vi "4 Axis - Wait for Arrival.vi"(4 "error in (no error)":errorcluster, 7 "Controller Reference In":refnum<k7>) -> (0 "error out":errorcluster, 3 "Controller Reference out":refnum<k7>)   [LabVIEW 2015]
doc: "Waits for all 4 Axis to arrive at their set Target Positions."
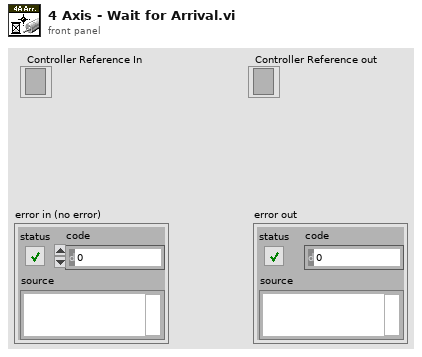
[diagram p1: front panel]
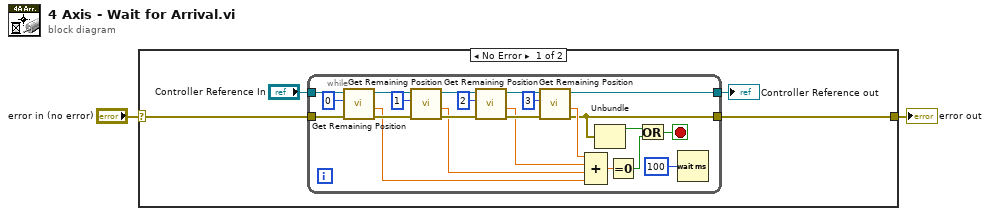
[diagram p0: block diagram]
diagram:
  n1 = case shown="No Error" "error in (no error)" {
    selector: "error in (no error)" -> [w3 w30]
    tunnel: [w4 w30] -> w2
    frame No Error {
      n2 = while {
        tunnel: "Controller Reference In" -> [w29]
        tunnel: [w17] -> w5
        tunnel: w3 -> [w28]
        tunnel: [w11] -> w4
        stop <- w8 stop-if-true
        n3 = call "Get Remaining Position.vi"("error in (no error)"=w28, "Axis In"=i16 0, "Controller Reference In"=w29) -> ("error out"=w24:errorcluster, "Position Remaining"=w13:sgl, "Controller Reference Out"=w22:refnum<k7>)  [unwired: 1 in, 1 out]
        n4 = call "Get Remaining Position.vi"("error in (no error)"=w24, "Axis In"=i16 1, "Controller Reference In"=w22) -> ("error out"=w20:errorcluster, "Position Remaining"=w14:sgl, "Controller Reference Out"=w21:refnum<k7>)  [unwired: 1 in, 1 out]
        n5 = call "Get Remaining Position.vi"("error in (no error)"=w20, "Axis In"=i16 2, "Controller Reference In"=w21) -> ("error out"=w19:errorcluster, "Position Remaining"=w15:sgl, "Controller Reference Out"=w18:refnum<k7>)  [unwired: 1 in, 1 out]
        n6 = call "Get Remaining Position.vi"("error in (no error)"=w19, "Axis In"=i16 3, "Controller Reference In"=w18) -> ("error out"=w11:errorcluster, "Position Remaining"=w16:sgl, "Controller Reference Out"=w17:refnum<k7>)  [unwired: 1 in, 1 out]
        n7 = Compound Arithmetic op=ADD(w16, w15, w14, w13) -> (w12:sgl)
        n8 = Unbundle(w11) -> ("status"=w10:bool)  [unwired: 2 out]
        n9 = Equal To 0?(x=w12) -> (x = 0?=w9:bool)
        n10 = Or(x=w10, y=w9) -> (x .or. y?=w8:bool)
        n11 = Wait (ms)(milliseconds to wait=u32 100) -> ()  [unwired: 1 out]
      }
      "Controller Reference out" <- w5
    }
    frame Error {
    }
  }
  "error out" <- w2
